vi "Entry Console View.vi"(8 "error in (no error)":errorcluster, 11 "View Model":T2) -> (0 "error out":errorcluster)   [LabVIEW 2017]
doc: "The interface via which the user selects the car wash options to be executed by the Car Wash Controller.\n[Covers: UI2]"
uses:
  View Model/Controls/View Model.ctl
  View Model/Controls/Shared Model.ctl
  Error Handler/Controls/Error Model.ctl
  Error Handler/Controls/Error Message.ctl
  Error Handler/Controls/Error Level.ctl
  Configuration/Controls/Database Model.ctl
  Configuration/Controls/Database Message.ctl
  Configuration/Controls/Database Command.ctl
  Configuration/Controls/Database Overhead.ctl
  Configuration/Controls/Database Status.ctl
  Configuration/Controls/Database Record.ctl
  Controller/Controls/CNTRLR - Model.ctl
  Controller/Controls/CNTRLR - Message.ctl
  Controller/Controls/CNTRLR - Command.ctl
  Controller/Controls/CNTRLR - Overhead.ctl
  Controller/Controls/CNTRLR - Position.ctl
  Controller/Controls/CNTRLR - State.ctl
  Controls/Entry - Wash Steps.ctl
  Controls/Entry - UI References.ctl
panel:
  in  "Start Wash":bool
  in  "Wash Steps":T1
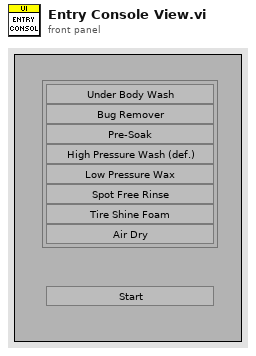
[diagram p1: front panel]
types:
  T1 = typedef "Entry - Wash Steps.ctl" = cluster{"Under Body Wash":bool, "Bug Remover":bool, "Pre-Soak":bool, "High Pressure Wash":bool, "Low Pressure Wax":bool, "Spot Free Rinse":bool, "Tire Shine Foam":bool, "Air Dry":bool}
  T2 = typedef "View Model.ctl" = cluster{"Shared Model":T3, "Error Model":T4, "DB Model":T5, "CNTRLR Model":T6}
  T3 = typedef "Shared Model.ctl" = cluster{"Stop":refnum<user-event>, "Stop DVR":refnum<data-value>}
  T4 = typedef "Error Model.ctl" = cluster{"Error Message":refnum<user-event>}
  T5 = typedef "Database Model.ctl" = cluster{"DB Message":refnum<user-event>, "DB Overhead DVR":refnum<data-value>}
  T6 = typedef "CNTRLR - Model.ctl" = cluster{"Message":refnum<user-event>, "Overhead DVR":refnum<data-value>}
  T7 = typedef "Entry - UI References.ctl" = cluster{"Wash Steps":refnum<vi>, "Start":refnum<vi>}
  T8 = enum8{"Enabled", "Disabled", "Disabled and Grayed Out"}
  T9 = typedef "CNTRLR - Command.ctl" = enum16{"Idle", "Start Car Wash", "Error", "Stop"}
  T10 = typedef "CNTRLR - State.ctl" = enum16{"Initial", "Wait for Start", "Start State", "Wait for Vehicle Position", "Wash Step Execution", "Wash Step/Cycle Complete", "Wash Exit", "Wash Abort/Terminate"}
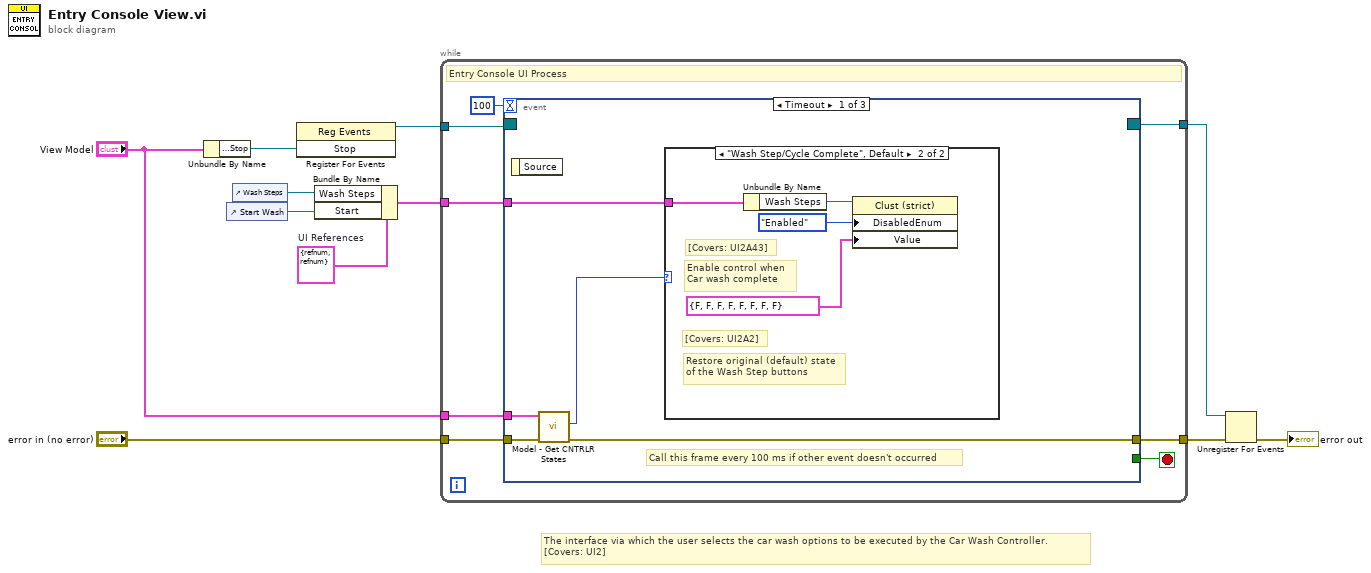
[diagram p0: block diagram]
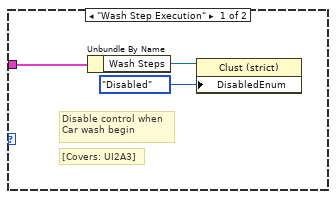
[diagram p2: hidden frame]
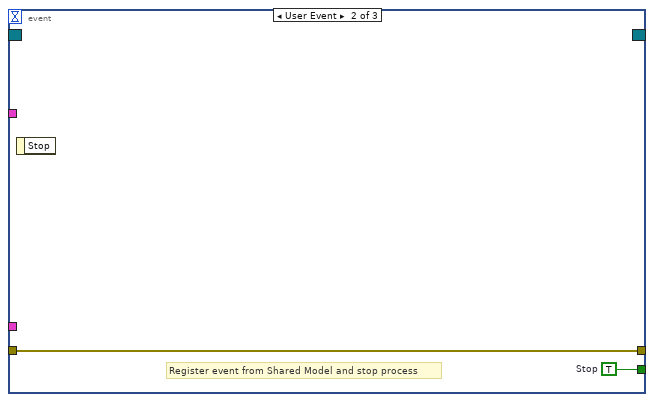
[diagram p3: hidden frame]
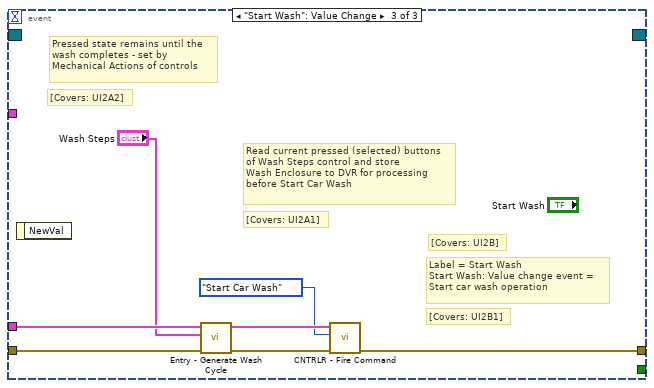
[diagram p4: hidden frame]
diagram:
  w5 = T7 {"Wash Steps"=refnum, "Start"=refnum}  # UI References
  # "The interface via which the user selects the car wash options to be executed by the Car Wash Controller.\n[Covers: UI2]"
  n1 = Unbundle By Name("View Model") -> ("Shared Model.Stop"=w11:refnum<user-event>)
  n2 = control-ref of="Start Wash"() -> (w3:refnum<vi>)
  n3 = control-ref of="Wash Steps"() -> (w4:refnum<vi>)
  n4 = register-events(w11) -> (reference out=w10:refnum<event-registration>)  [unwired: 2 in, 1 out]
  n5 = Bundle By Name(cluster=w5, "Wash Steps"=w4, "Start"=w3) -> (w2:T7)
  n6 = while {
    tunnel: w10 -> [w19]
    tunnel: "error in (no error)" -> [w18]
    tunnel: [w17] -> w8
    tunnel: [w14] -> w9
    tunnel: "View Model" -> [w12]
    tunnel: w2 -> [w13]
    stop <- w15 stop-if-true
    # "Entry Console UI Process"
    n7 = event shown="[0] Timeout" {
      selector: w19 -> [_ _ _]
      dyn-events: [_ _ _] -> w14
      timeout: 100 -> [_ _ _]
      tunnel: w18 -> [w24 w32 w40]
      tunnel: [w23 w32 w35] -> w17
      tunnel: [_ w33 _] -> w15
      tunnel: w13 -> [w20 _ _]
      tunnel: w12 -> [w22 _ w39]
      event Timeout {
        # "Call this frame every 100 ms if other event doesn't occurred"
        n8 = event-data() -> ()  [unwired: 1 in, 1 out]
        n9 = call "Model - Get CNTRLR States.vi"("error in (no error)"=w24, "View Model"=w22) -> ("error out"=w23:errorcluster, "Current State"=w21:T10)  [unwired: 6 in, 2 out]
        n10 = case shown="\"Wash Step/Cycle Complete\", Default" w21 {
          tunnel: w20 -> [w26 w30]
          frame "Wash Step Execution" {
            # "[Covers: UI2A3]"
            # "Disable control when\nCar wash begin"
            n11 = Unbundle By Name(w26) -> ("Wash Steps"=w27:refnum<vi>)
            n12 = property class="Clust (strict)"(reference=w27, "DisabledEnum"=T8."Disabled" ("Disabled")) -> ()  [unwired: 1 in, 2 out]
          }
          frame "Wash Step/Cycle Complete", Default {
            # "[Covers: UI2A2]"
            # "Restore original (default) state\nof the Wash Step buttons"
            # "[Covers: UI2A43]"
            # "Enable control when\nCar wash complete"
            n13 = Unbundle By Name(w30) -> ("Wash Steps"=w31:refnum<vi>)
            n14 = property class="Clust (strict)"(reference=w31, "DisabledEnum"=T8."Enabled" ("Disabled"), "Value"=T1 {"Under Body Wash"=FALSE, "Bug Remover"=FALSE, "Pre-Soak"=FALSE, "High Pressure Wash"=FALSE, "Low Pressure Wax"=FALSE, "Spot Free Rinse"=FALSE, "Tire Shine Foam"=FALSE, "Air Dry"=FALSE}) -> ()  [unwired: 1 in, 2 out]
          }
        }
      }
      event User Event {
        w33 = TRUE  # Stop
        # "Register event from Shared Model and stop process"
        n15 = event-data() -> ()  [unwired: 1 in, 1 out]
      }
      event "Start Wash": Value Change {
        # "[Covers: UI2B1]"
        # "[Covers: UI2B]"
        # "Label = Start Wash\nStart Wash: Value change event = \nStart car wash operation"
        # "[Covers: UI2A1]"
        # "Read current pressed (selected) buttons\nof Wash Steps control and store \nWash Enclosure to DVR for processing\nbefore Start Car Wash"
        # "[Covers: UI2A2]"
        # "Pressed state remains until the \nwash completes - set by\nMechanical Actions of controls"
        n16 = event-data() -> ()  [unwired: 1 in, 1 out]
        n17 = call "Entry - Generate Wash Cycle.vi"("error in (no error)"=w40, "Wash Steps"="Wash Steps", "View Model"=w39) -> ("error out"=w37:errorcluster, "View Model"=w36:T2)  [unwired: 7 in]
        n18 = call "CNTRLR - Fire Command.vi"("error in (no error)"=w37, "CMD"=CNTRLR_-_Command."Start Car Wash", "View Model"=w36) -> ("error out"=w35:errorcluster)  [unwired: 8 in]
      }
    }
  }
  n19 = Unregister For Events(event registration refnum=w9, error in=w8) -> (error out=→"error out":errorcluster)
